vi "plc read float.vi"(8 "error in":errorcluster, 10 "Timeout (ms)":i32=1000, 11 "addr,tag":T1 {"DataSocket Reference"."OnStatusUpdated" format="%.0x"; "DataSocket Reference"."OnDataUpdated" format="%.0x"}) -> (0 "error out":errorcluster, 3 "value":sgl)   [LabVIEW 2018]
uses:
  05.UserVI's/type defs/plc path and tag.ctl
  <vilib>/Platform/dataskt.llb/DataSocket Reference Type.ctl
  <vilib>/ethernetip/ethernetip.llb/EthernetIP Tag Read REAL.vi
  <vilib>/ethernetip/ethernetip.lvlib
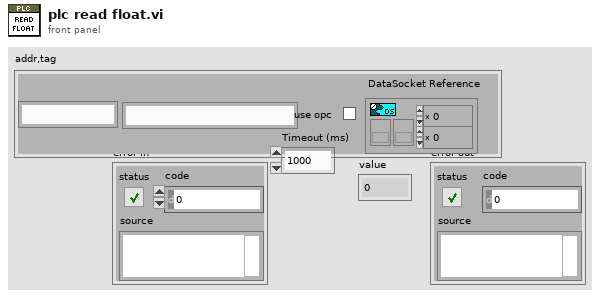
[diagram p1: front panel]
types:
  T1 = typedef "plc path and tag.ctl" = cluster{"Tag Name":string, "Network Path":string, "use opc":bool, "DataSocket Reference":T2}
  T2 = typedef "DataSocket Reference Type.ctl" = cluster{"CWDSLib._DCWDataSocket":refnum<k7>, "CWDSLib._DCWData":refnum<k7>, "OnDataUpdated":u32, "OnStatusUpdated":u32}
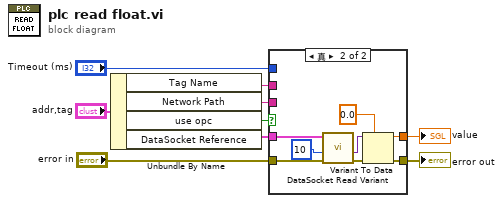
[diagram p0: block diagram]
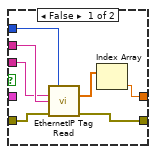
[diagram p2: hidden frame]
diagram:
  n1 = Unbundle By Name("addr,tag") -> ("Tag Name"=w7:string, "Network Path"=w6:string, "use opc"=w3:bool, "DataSocket Reference"=w2:T2)
  n2 = case shown="真" w3 {
    tunnel: "error in" -> [w16 w23]
    tunnel: [w15 w20] -> w8
    tunnel: w7 -> [w14 _]
    tunnel: w6 -> [w13 _]
    tunnel: [w12 w18] -> w1
    tunnel: "Timeout (ms)" -> [w10 _]
    tunnel: w2 -> [_ w22]
    frame False {
      n3 = call-poly <vilib>:"EthernetIP Tag Read.vi"("Timeout (ms)"=w10, "Network Path"=w13, "Tag Name"=w14, "error in"=w16) -> ("Data"=w11:sgl[], "error out"=w15:errorcluster)  [unwired: 9 in, 1 out]
      n4 = Index Array(array=w11) -> (element=w12:sgl)  [unwired: 1 in]
    }
    frame True {
      n5 = call <vilib>:"DataSocket Read Variant.vi"("error in (no error)"=w23, "Timeout (1000 ms)"=10, "DataSocket Reference In"=w22) -> ("error out"=w21:errorcluster, "Data"=w19:variant)  [unwired: 2 in, 3 out]
      n6 = Variant To Data(error in=w21, type=sgl 0.0 ("value"), Variant=w19) -> (data=w18:sgl, error out=w20:errorcluster)
    }
  }
  "error out" <- w8
  "value" <- w1
